vi "Read Status Source.vi"(8 "error in (no error)":errorcluster, 11 "VisaComms in":refnum<class "VisaComms.lvclass">) -> (0 "error out":errorcluster, 2 "Status Source":T1, 3 "VisaComms out":refnum<class "VisaComms.lvclass">)   [LabVIEW 2024, in "CTI.lvlib" / "VisaComms.lvclass"]
uses:
  VisaComms.lvclass
  Status Source.ctl
  VisaComms.lvclass/VisaComms.ctl
  Clean Visa Errors.vi
  CTI.lvlib
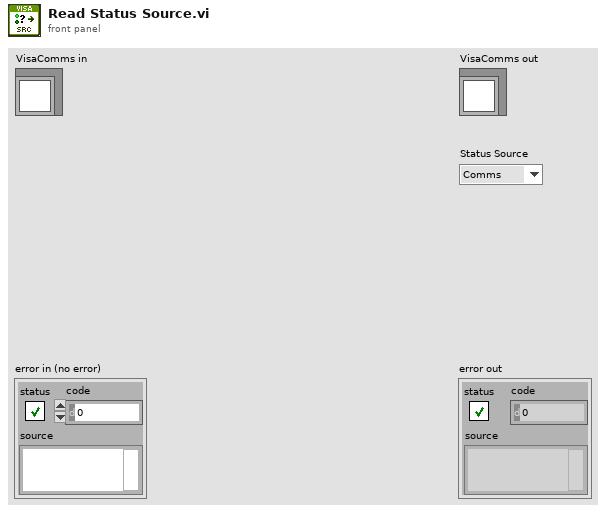
[diagram p1: front panel]
types:
  T1 = typedef "CTI.lvlib/Status Source.ctl" = enum16{"Comms", "User"}
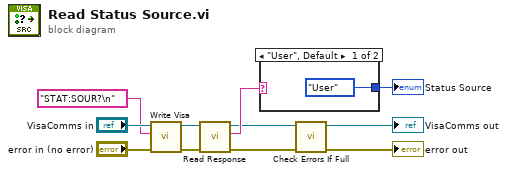
[diagram p0: block diagram]
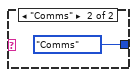
[diagram p2: hidden frame]
diagram:
  n1 = call "Write Visa.vi"("error in (no error)"="error in (no error)", "write buffer"="STAT:SOUR?\n" ("format string"), "VisaComms in"="VisaComms in") -> ("error out"=w10:errorcluster, "VisaComms out"=w6:refnum<class "VisaComms.lvclass">)  [unwired: 6 in, 1 out]
  n2 = call "Read Response.vi"("error in (no error)"=w10, "VisaComms in"=w6) -> ("error out"=w7:errorcluster, "Response"=w5:string, "VisaComms out"=w2:refnum<class "VisaComms.lvclass">)  [unwired: 6 in, 1 out]
  n3 = case shown="\"User\", Default" w5 {
    tunnel: [Status_Source."User" ("Status Source") Status_Source."Comms" ("Status Source")] -> w4
    frame "User", Default {
    }
    frame "Comms" {
    }
  }
  "Status Source" <- w4
  n4 = call "Check Errors If Full.vi"("error in (no error)"=w7, "VisaComms in"=w2) -> ("error out"=→"error out":errorcluster, "VisaComms out"=→"VisaComms out":refnum<class "VisaComms.lvclass">)  [unwired: 8 in]
